vi "create_standardized_delay_array.vi"(4 "delay array":dbl[](array[numeric]), 5 "resolution":i32=100) -> (1 "standardize array":dbl[](array[numeric]), 2 "multiplier":i32)   [LabVIEW 2011]
doc: "creates a standardize array that can be easily displayed no matter what the time unit in the array is. covers second to nanoseconds."
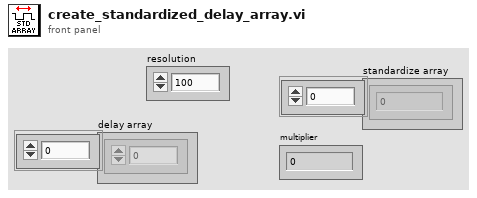
[diagram p1: front panel]
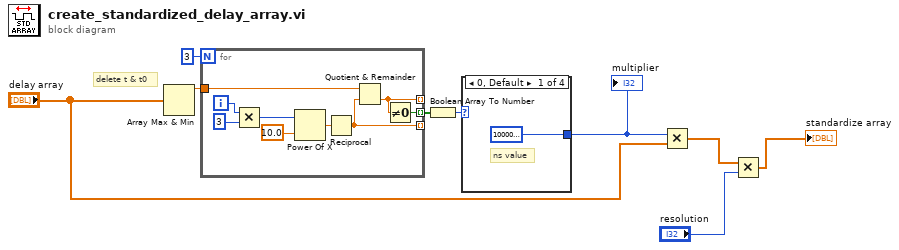
[diagram p0: block diagram]
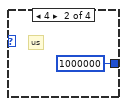
[diagram p2: hidden frame]
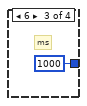
[diagram p3: hidden frame]
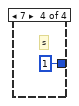
[diagram p4: hidden frame]
diagram:
  # "delete t & t0"
  n1 = Array Max & Min(array="delay array") -> (max value=w6:dbl)  [unwired: 3 out]
  n2 = for {
    N: 3 -> [_]
    tunnel: w6 -> [w15]
    tunnel: [w10] -> _ mode=indexing
    tunnel: [w14] -> _ mode=indexing
    tunnel: [w13] -> w8 mode=indexing
    i -> [w12]
    n3 = Multiply(x=w12, y=3) -> (x*y=w16:i32)
    n4 = Power Of X(1:10.0 ("x"), 2:w16) -> (0:w11:dbl)
    n5 = Reciprocal(x=w11) -> (1/x=w10:dbl)
    n6 = Quotient & Remainder(x=w15, y=w10) -> (floor(x/y)=w14:dbl)  [unwired: 1 out]
    n7 = Not Equal To 0?(x=w14) -> (x != 0?=w13:bool)
  }
  n8 = Boolean Array To Number(Boolean array=w8) -> (number=w7:u32)
  n9 = case shown="0, Default" w7 {
    tunnel: [1000000000 1000000 1000 1] -> w1
    frame 0, Default {
      # "ns value"
    }
    frame 4 {
      # "us"
    }
    frame 6 {
      # "ms"
    }
    frame 7 {
      # "s"
    }
  }
  "multiplier" <- w1
  n10 = Multiply(x=w1, y="delay array") -> (x*y=w4:dbl[])
  n11 = Multiply(x=w4, y="resolution") -> (x*y=→"standardize array":dbl[])
